vi "parse by space_v2.vi"(8 "error in (no error)":errorcluster, 11 "String":string) -> (0 "error out":errorcluster, 3 "Array":string[](array[string]))   [LabVIEW 2016]
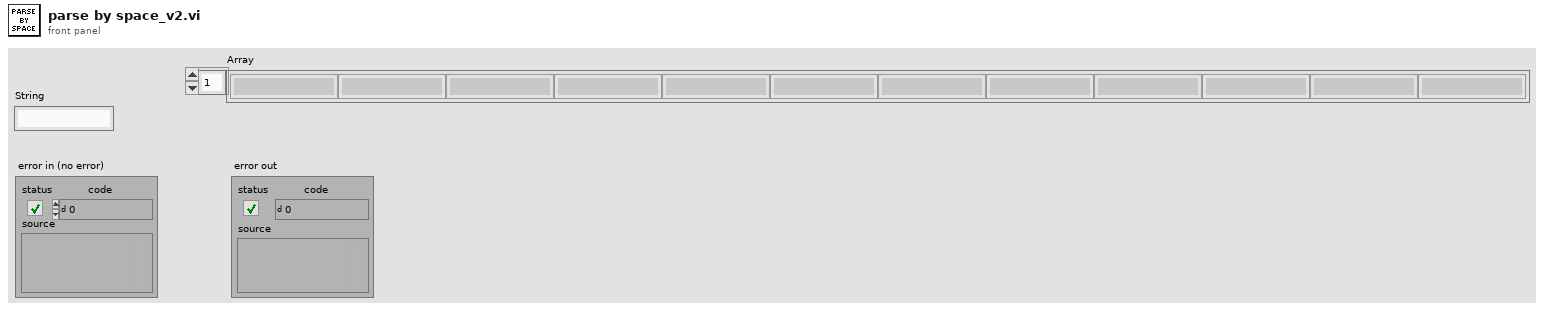
[diagram p1: front panel]
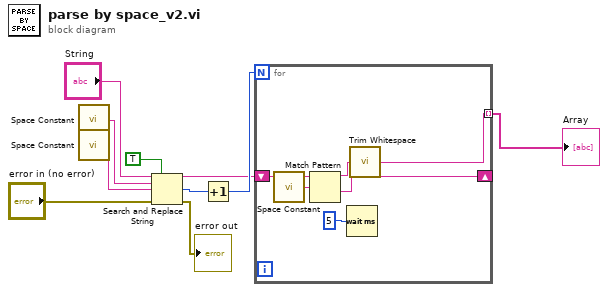
[diagram p0: block diagram]
diagram:
  n1 = call <vilib>:"Space Constant.vi"() -> ("String"=w9:string)
  n2 = call <vilib>:"Space Constant.vi"() -> ("String"=w8:string)
  n3 = Search and Replace String(replace all?=TRUE ("ignore case? (F)"), input string="String", search string=w9, replace string=w8, error in="error in (no error)") -> (result string=w4:string, number of replacements=w6:i32, error out=→"error out":errorcluster)  [unwired: 3 in, 1 out]
  n4 = Increment(x=w6) -> (x+1=w5:i32)
  n5 = for {
    N: w5 -> [_]
    shift-right: [w12] -> _
    shift-left: w4 -> [w16]
    tunnel: [w11] -> w1 mode=indexing
    n6 = call <vilib>:"Space Constant.vi"() -> ("String"=w15:string)
    n7 = Match Pattern(string=w16, regular expression=w15) -> (before substring=w13:string, after substring=w12:string)  [unwired: 1 in, 2 out]
    n8 = Wait (ms)(milliseconds to wait=u32 5) -> ()  [unwired: 1 out]
    n9 = call <vilib>:"Trim Whitespace.vi"("string"=w13) -> ("trimmed string"=w11:string)  [unwired: 1 in]
  }
  "Array" <- w1
